vi "WinCI File Status.vi"(8 "error in (no error)":errorcluster, 10 "files":path[](array[path]), 11 "source control reference in":T2) -> (0 "error out":errorcluster, 1 "file status":T1[](array[typedef]), 2 "status message":string, 3 "source control reference out":T2, 4 "files status flags":i32[](array[numeric]))   [LabVIEW 2017, in "NI_SCC_WinCI.lvlib"]
uses:
  <vilib>/SourceControl/Providers/WinCI/NI_SCC_WinCI.lvlib
  <vilib>/SourceControl/sccapi/SCCAPI Refnum.ctl
  <vilib>/SourceControl/sccapi/SCCAPI SCC File Status.ctl
  <vilib>/SourceControl/sccapi/NI_SCC.lvlib
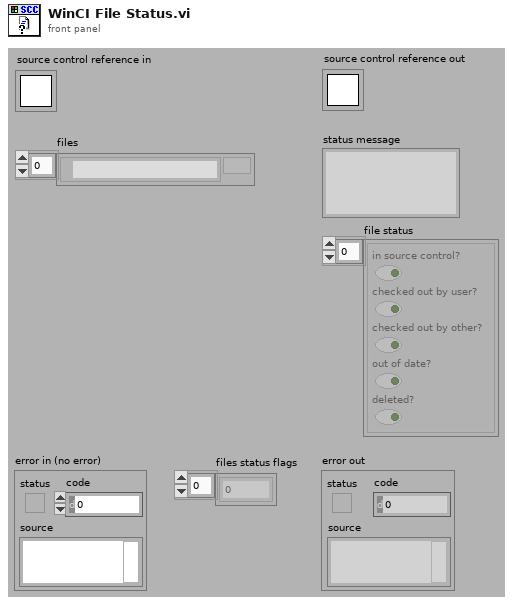
[diagram p1: front panel]
types:
  T1 = typedef "NI_SCC.lvlib/SCCAPI SCC File Status.ctl" = cluster{"in source control?":bool, "checked out by user?":bool, "checked out by other?":bool, "out of date?":bool, "deleted?":bool}
  T2 = typedef "NI_SCC.lvlib/SCCAPI Refnum.ctl" = refnum<k1>
  T3 = typedef "NI_SCC_WinCI.lvlib/WinCI SCC File Status.ctl" = cluster{"valid status?":bool, "scc status":cluster{"source controlled":bool, "checked out":bool, "checked out by other":bool, "exclusively checked out":bool, "checked out by multiple":bool, "out of date":bool, "deleted":bool, "locked":bool, "merged":bool, "shared":bool, "pinned":bool, "modified":bool, "checked out by user":bool}}
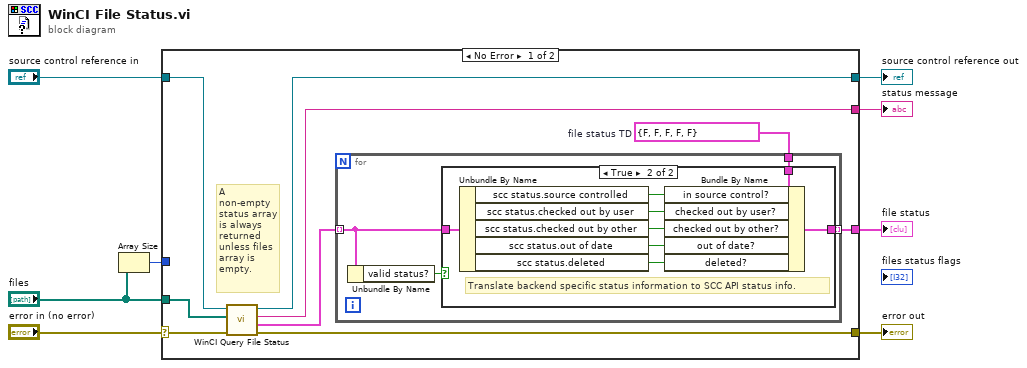
[diagram p0: block diagram]
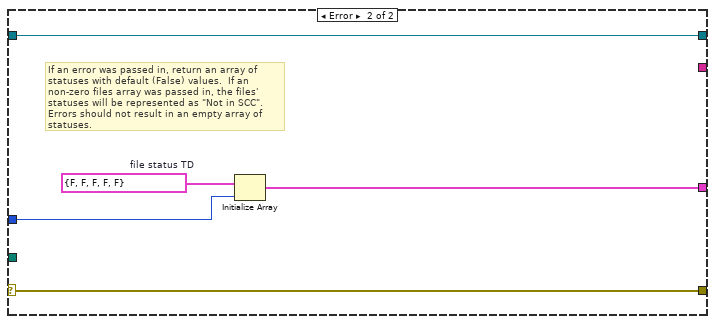
[diagram p3: hidden frame]
diagram:
  n1 = Array Size(array="files") -> (size(s)=w1:i32)
  n2 = case shown="No Error" "error in (no error)" {
    selector: "error in (no error)" -> [w10 w35]
    tunnel: [w11 w35] -> w7
    tunnel: "source control reference in" -> [w15 w34]
    tunnel: [w13 _] -> w5
    tunnel: "files" -> [w9 _]
    tunnel: [w14 w34] -> w4
    tunnel: [w16 w32] -> w3
    tunnel: w1 -> [_ w33]
    frame No Error {
      w17 = T1 {"in source control?"=FALSE, "checked out by user?"=FALSE, "checked out by other?"=FALSE, "out of date?"=FALSE, "deleted?"=FALSE}  # file status TD
      # "A non-empty status array  is always returned unless files array is empty."
      n3 = call <vilib>:"WinCI Query File Status.vi"("error in (no error)"=w10, "files"=w9, "source control reference in"=w15) -> ("error out"=w11:errorcluster, "file status"=w12:T3[], "status message"=w13:string, "source control reference out"=w14:T2)  [unwired: 5 out]
      n4 = for {
        tunnel: w12 -> [w20] mode=indexing
        tunnel: w17 -> [w19]
        tunnel: [w18] -> w16 mode=indexing
        n5 = Unbundle By Name(w20) -> ("valid status?"=w21:bool)
        n6 = case shown="True" w21 {
          tunnel: w20 -> [_ w30]
          tunnel: w19 -> [w22 w29]
          tunnel: [w22 w28] -> w18
          frame False {
          }
          frame True {
            # "Translate backend specific status information to SCC API status info."
            n7 = Unbundle By Name(w30) -> ("scc status.source controlled"=w27:bool, "scc status.checked out by user"=w26:bool, "scc status.checked out by other"=w25:bool, "scc status.out of date"=w24:bool, "scc status.deleted"=w23:bool)
            n8 = Bundle By Name(cluster=w29, "in source control?"=w27, "checked out by user?"=w26, "checked out by other?"=w25, "out of date?"=w24, "deleted?"=w23) -> (w28:T1)
          }
        }
      }
    }
    frame Error {
      w31 = T1 {"in source control?"=FALSE, "checked out by user?"=FALSE, "checked out by other?"=FALSE, "out of date?"=FALSE, "deleted?"=FALSE}  # file status TD
      # "If an error was passed in, return an array of statuses with default (False) values.  If an non-zero files array was passed in, the files' statuses will be represented as \"Not in SCC\".  Errors should not result in an empty array of statuses."
      n9 = Initialize Array(w31, w33) -> (w32:T1[])
    }
  }
  "error out" <- w7
  "status message" <- w5
  "source control reference out" <- w4
  "file status" <- w3
